vi "Pre Launch Init.vi"(11 "Sequencer in":refnum<class "Sequencer.lvclass">) -> (0 "error out":errorcluster, 3 "Sequencer out":refnum<class "Sequencer.lvclass">)   [LabVIEW 2020, in "Sequencer.lvlib" / "Sequencer.lvclass"]
doc: "(<B>Filename</B>: Actor Framework.lvlib:Actor.lvclass:Pre Launch Init.vi)\n\nDefines behavior that occurs after the Launch Nested Actor method is invoked but before the actor's Actor Core method begins running.\n\nThis implementation launches the Sequencer Core."
uses:
  Sequencer.lvclass
  C:/Current projects/WS/PPL/HDH.Actor Framework.Core.Actor.lvlibp/1abvi3w/vi.lib/ActorFramework/Actor/Actor.lvclass
  Sequencer.lvclass/Sequencer.ctl
  PPL/HDH.Actor Framework.Core.Actor.lvlibp/1abvi3w/vi.lib/ActorFramework/Actor/Actor.lvclass
  Sequencer Core/Sequencer Core.lvclass
  PPL/HDH.Actor Framework.Core.Utility.lvlibp
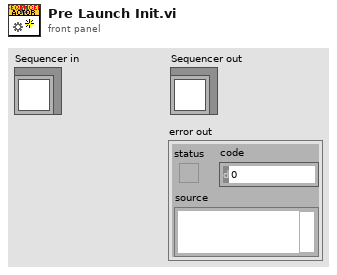
[diagram p1: front panel]
types:
  T1 = typedef "Semaphore RefNum" = refnum<k1>
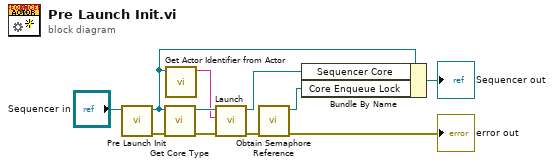
[diagram p0: block diagram]
diagram:
  n1 = call-parent "Pre Launch Init.vi"("Actor in"="Sequencer in") -> ("error out"=w8:errorcluster, "Actor out"=w1:refnum<class "Sequencer.lvclass">)  [unwired: 9 in]
  n2 = call-dynamic "Get Core Type.vi"("error in (no error)"=w8, "Sequencer in"=w1) -> ("error out"=w7:errorcluster, "Sequencer Core out"=w9:refnum<class "Sequencer Core.lvclass">)  [unwired: 8 in]
  n3 = call "Get Actor Identifier from Actor.vi"("Actor in"=w1) -> ("Actor ID string out"=w2:string)  [unwired: 9 in, 1 out]
  n4 = call "Launch.vi"("error in (no error)"=w7, "Enqueuer ID string in"=w2, "Sequencer Core in"=w9) -> ("error out"=w5:errorcluster, "Sequencer Core out"=w6:refnum<class "Sequencer Core.lvclass">)  [unwired: 7 in]
  n5 = call <vilib>:"Obtain Semaphore Reference.vi"("error in (no error)"=w5) -> ("error out"=→"error out":errorcluster, "semaphore"=w3:T1)  [unwired: 4 in, 1 out]
  n6 = Bundle By Name(cluster=w1, "Sequencer Core"=w6, "Core Enqueue Lock"=w3) -> (→"Sequencer out":refnum<class "Sequencer.lvclass">)
